vi "niHWS Write Digital WDT.vi"(8 "error in (no error)":errorcluster, 10 "digital waveform":digitalwaveform(waveform), 11 "waveform reference in":u32) -> (0 "error out":errorcluster, 3 "waveform reference out":u32)   [LabVIEW 2020]
doc: "Writes digital waveform data into the file beginning at the current read/write position.\n\nThis VI is only supported in LabVIEW 7.0 and later."
uses:
  niHWS Set Wfm DBL Attribute ID.ctl
  DWDT Uncompress Digital.vi
  nihwsu.dll
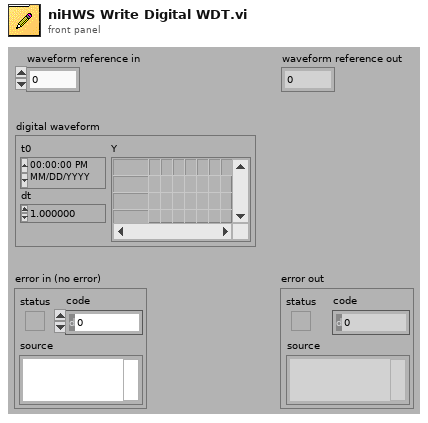
[diagram p1: front panel]
types:
  T1 = typedef "niHWS Set Wfm DBL Attribute ID.ctl" = u32
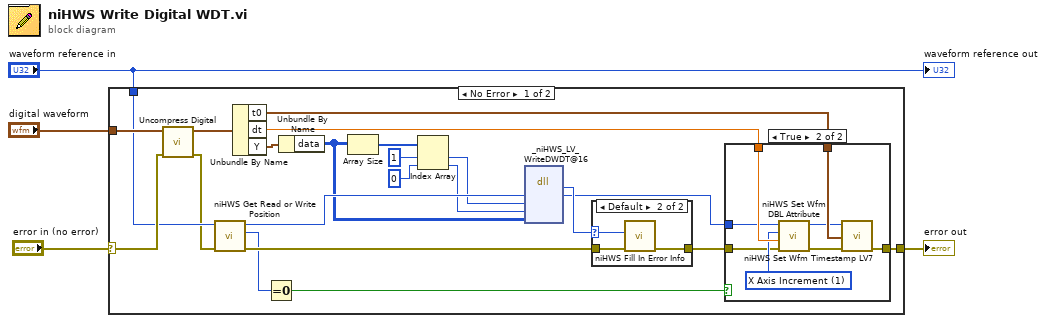
[diagram p0: block diagram]
diagram:
  n1 = case shown="No Error" "error in (no error)" {
    selector: "error in (no error)" -> [w19 w40]
    tunnel: [w13 w40] -> w4
    tunnel: "waveform reference in" -> [w17 _]
    tunnel: "digital waveform" -> [w21 _]
    frame No Error {
      n2 = call-poly "Uncompress Digital.vi"("error in (no error)"=w19, "compressed digital waveform"=w21) -> ("error out"=w16:errorcluster, "uncompressed digital waveform"=w20:digitalwaveform)  [unwired: 8 in]
      n3 = call "niHWS Get Read or Write Position.vi"("waveform reference in"=w17, "error in (no error)"=w16) -> ("waveform reference out"=w18:u32, "position"=w12:u32, "error out"=w15:errorcluster)  [unwired: 6 in]
      n4 = Unbundle By Name(w20) -> ("t0"=w8:timestamp, "dt"=w9:dbl, "Y"=w23:digitaldata)
      n5 = Equal To 0?(x=w12) -> (x = 0?=w11:bool)
      n6 = Unbundle By Name(w23) -> ("data"=w5:u8[][])
      n7 = Array Size(array=w5) -> (size(s)=w26:i32[])
      n8 = Index Array(array=w26, index #1=1 ("index"), index #2=0 ("index")) -> (element #1=w7:i32, element #2=w6:i32)
      n9 = dll-call lib="nihwsu.dll" fn="_niHWS_LV_WriteDWDT@16"("wfmReference"=w18, "numSignals"=w7, "numSamples"=w6, "wfmData"=w5) -> (w22:i32, "wfmReference"=w10:u32)  [unwired: 6 in, 2 out]
      n10 = case shown="Default" w22 {
        selector: w22 -> [_ w37]
        tunnel: [w36 w38] -> w14
        tunnel: w15 -> [w36 w39]
        frame 0 {
        }
        frame Default {
          n11 = call "niHWS Fill In Error Info.vi"("error in (no error)"=w39, "status code"=w37) -> ("error out"=w38:errorcluster)  [unwired: 9 in]
        }
      }
      n12 = case shown="True" w11 {
        tunnel: w9 -> [_ w34]
        tunnel: w8 -> [_ w33]
        tunnel: [w27 w32] -> w13
        tunnel: w10 -> [_ w29]
        tunnel: w14 -> [w27 w28]
        frame False {
        }
        frame True {
          w30 = T1 1 items=["X Axis Start"=0, "X Axis Increment"=1, "Y Axis Minimum"=3, "Y Axis Maximum"=4] ("Attribute ID")
          n13 = call "niHWS Set Wfm DBL Attribute.vi"("error in (no error)"=w28, "attribute value"=w34, "attribute ID"=w30, "waveform reference in"=w29) -> ("error out"=w35:errorcluster, "waveform reference out"=w31:u32)  [unwired: 6 in]
          n14 = call "niHWS Set Wfm Timestamp LV7.vi"("error in (no error)"=w35, "waveform timestamp"=w33, "waveform reference in"=w31) -> ("error out"=w32:errorcluster)  [unwired: 7 in, 1 out]
        }
      }
    }
    frame Error {
    }
  }
  "error out" <- w4
  "waveform reference out" <- "waveform reference in"
